vi "Generate Shutdown Event.vi"(8 "error in (no error)":errorcluster) -> (0 "error out":errorcluster)   [LabVIEW 2018, in "Launcher.lvlib"]
uses:
  Launcher.lvlib
  Shutdown Event FGV Command.ctl
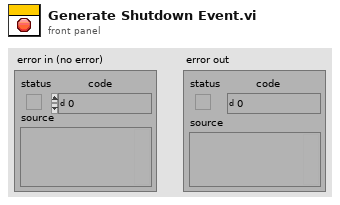
[diagram p1: front panel]
types:
  T1 = typedef "Launcher.lvlib/Shutdown Event FGV Command.ctl" = enum16{"Create Event", "Get Event Ref", "Release Event"}
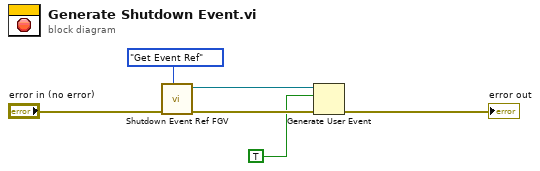
[diagram p0: block diagram]
diagram:
  n1 = call "Shutdown Event Ref FGV.vi"("Command"=Shutdown_Event_FGV_Command."Get Event Ref", "error in (no error)"="error in (no error)") -> ("error out"=w3:errorcluster, "Shutdown"=w4:refnum<user-event>)  [unwired: 8 in]
  n2 = Generate User Event(user event=w4, event data cluster=TRUE ("event data"), error in=w3) -> (error out=→"error out":errorcluster)  [unwired: 1 in, 1 out]
